vi "read_attributes.vi"(8 "error in (no error)":errorcluster, 11 "DecisionTreeClassifier in":refnum<class "DecisionTreeClassifier.lvclass">) -> (0 "error out":errorcluster, 2 "attributes":T1, 3 "DecisionTreeClassifier out":refnum<class "DecisionTreeClassifier.lvclass">)   [LabVIEW 2020, in "DecisionTreeClassifier.lvclass"]
uses:
  DecisionTreeClassifier.lvclass
  Controls/decision_tree_classifier_attributes.ctl
  DecisionTreeClassifier.lvclass/DecisionTreeClassifier.ctl
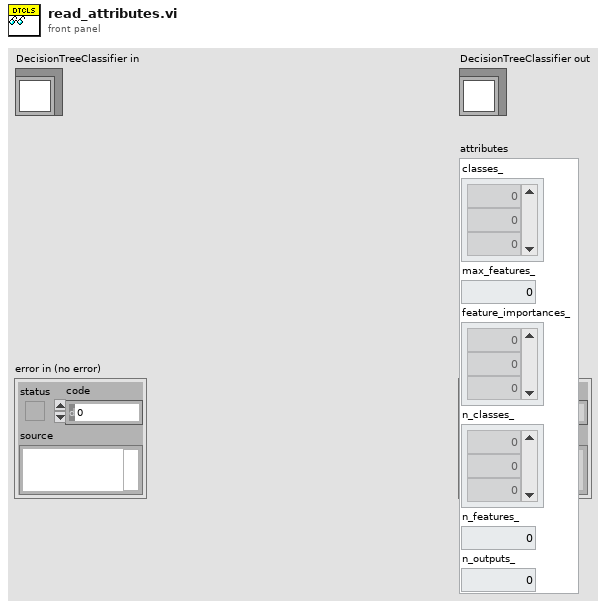
[diagram p1: front panel]
types:
  T1 = typedef "decision_tree_classifier_attributes.ctl" = cluster{"classes_":dbl[][], "max_features_":dbl, "feature_importances_":dbl[], "n_classes_":dbl[], "n_features_":dbl, "n_outputs_":dbl}
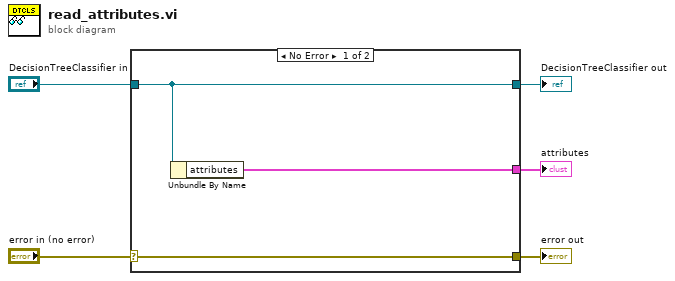
[diagram p0: block diagram]
diagram:
  n1 = case shown="No Error" "error in (no error)" {
    selector: "error in (no error)" -> [w8 w9]
    tunnel: [w8 w9] -> w4
    tunnel: [w7 w10] -> w2
    tunnel: "DecisionTreeClassifier in" -> [w7 w10]
    tunnel: [w6 _] -> w1
    frame No Error {
      n2 = Unbundle By Name(w7) -> ("attributes"=w6:T1)
    }
    frame Error {
    }
  }
  "error out" <- w4
  "DecisionTreeClassifier out" <- w2
  "attributes" <- w1
